vi "Read All Data.vi"() -> ()   [LabVIEW 2018]
doc: "This example returns data from the database you choose using the Connection Information, Username, and Password.\n\nA list of the database tables appears in the Table Names menu ring. You can then press the Get Data button to return all the data from the selected table into the Table Data indicator. The numbers of rows and columns in that table are also returned in the respective indicators. You press the Stop button when you are finished with the example. \n\nThis example was written to solve a unique problem associated with reading very large recordsets where the performance becomes slow from the use of a large amount of computer resources. SubVIs named DB Tools Select All Data and DB Tools Fetch Table Data have been optimized to use the least number of resources and thus provide the best performance when reading large recordsets."
uses:
  <vilib>/addons/database/Connection.llb/DB Tools Open Connec (String).vi
  <vilib>/addons/database/NI_Database_API.lvlib
panel:
  out "Columns":i32
  out "Rows":i32
  in  "Stop":bool
  in  "Table Names":u16(ring)
  out "Table Data":string[][](table)
  # "Overview: Demonstrates how to fetch individual tables from a database for display.\nRequirements: Database Connectivity Toolkit\nInstructions:\n1. Run this VI.\n2. Change the Table Names value to see the contents of a table displayed in the Table Data indicator.\n3. Click Stop to stop the VI."
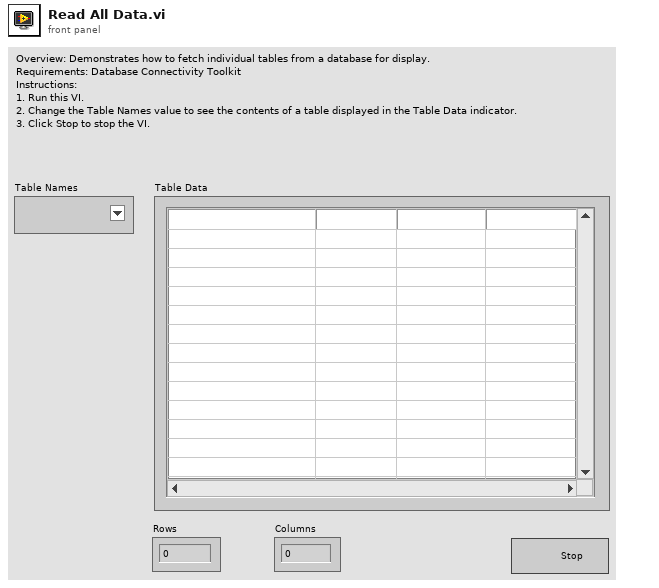
[diagram p1: front panel]
types:
  T1 = typedef "NI_Database_API.lvlib/Conn ObjectReference.ctl" = refnum<k1>
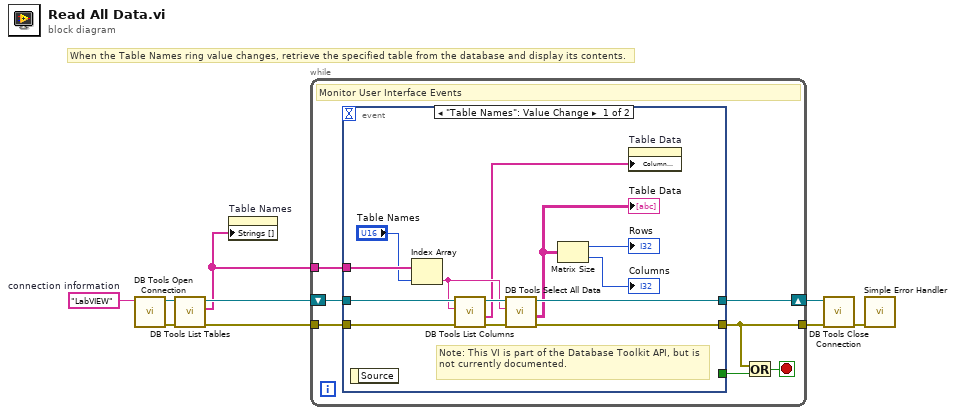
[diagram p0: block diagram]
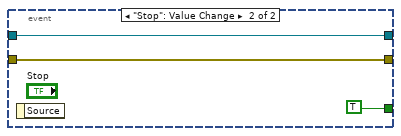
[diagram p2: hidden frame]
diagram:
  w1 = "LabVIEW"  # connection information
  # "When the Table Names ring value changes, retrieve the specified table from the database and display its contents."
  n1 = call-poly <vilib>:"DB Tools Open Connection.vi"("connection information"=w1) -> ("error out"=w5:errorcluster, "connection reference"=w6:T1)  [unwired: 7 in]
  n2 = call <vilib>:"DB Tools List Tables.vi"("error in (no error)"=w5, "connection reference"=w6) -> ("error out"=w4:errorcluster, "tables"=w2:string[], "connection reference out"=w3:T1)  [unwired: 3 in]
  n3 = property on="Table Names" class="Ring (strict)"("Strings []"=w2) -> ()  [unwired: 2 in, 2 out]
  n4 = while {
    tunnel: [w11] -> w7
    tunnel: w4 -> [w15]
    tunnel: w2 -> [w13]
    shift-right: [w16] -> w9
    shift-left: w3 -> [w14]
    stop <- w12 stop-if-true
    # "Monitor User Interface Events"
    n5 = event shown="[0] \"Table Names\": Value Change" {
      selector: _ -> [_ _]
      dyn-events: _ -> [_ _]
      timeout: _ -> [_ _]
      tunnel: [w29 w32] -> w16
      tunnel: w15 -> [w28 w31]
      tunnel: w14 -> [w27 w32]
      tunnel: w13 -> [w26 _]
      tunnel: [w19 w31] -> w11
      tunnel: [_ TRUE] -> w10
      event "Table Names": Value Change {
        # "Note: This VI is part of the Database Toolkit API, but is not currently documented."
        n6 = event-data() -> ()  [unwired: 1 in, 1 out]
        n7 = Index Array(array=w26, index="Table Names") -> (element=w22:string)
        n8 = call <vilib>:"DB Tools List Columns.vi"("error in (no error)"=w28, "table"=w22, "connection reference"=w27) -> ("error out"=w24:errorcluster, "columns"=w20:string[], "connection reference out"=w25:T1)  [unwired: 1 in, 1 out]
        n9 = call <vilib>:"DB Tools Select All Data.vi"("error in (no error)"=w24, "table"=w22, "connection reference"=w25) -> ("error out"=w19:errorcluster, "data"=w23:string[][], "connection reference out"=w29:T1)  [unwired: 3 in]
        "Table Data" <- w23
        n10 = Matrix Size(0:w23) -> (1:→"Rows":i32, 2:→"Columns":i32)
        n11 = property on="Table Data" class="Tbl (strict)"("Column Header Strings[]"=w20) -> ()  [unwired: 2 in, 2 out]
      }
      event "Stop": Value Change {
        n12 = event-data() -> ()  [unwired: 1 in, 1 out]
      }
    }
    n13 = Or(x=w11, y=w10) -> (x .or. y?=w12:bool)
  }
  n14 = call <vilib>:"DB Tools Close Connection.vi"("error in (no error)"=w7, "connection reference"=w9) -> ("error out"=w8:errorcluster)  [unwired: 5 in]
  n15 = call <vilib>:"Simple Error Handler.vi"("error in (no error)"=w8) -> ()  [unwired: 4 in, 5 out]
